vi "MagX Upload File.vi"(2 "Log File":path=path "C:/Data/April_2019/042419/sp0006_042419.tdms", 3 "Lab notebook entry":string, 4 "Append to Wiki":bool, 5 "Add-on storage":T1, 6 "Station":string="Cell_3", 7 "Create Markdown":bool, 8 "error in":errorcluster, 9 "Experiment ID":string, 10 "Log server":string="magx.lanl.gov", 11 "File name":path=path "C:/Data/April_2019/042419/sp0006_042419.tdms") -> (0 "error out":errorcluster)   [LabVIEW 2024]
uses:
  Add-on Storage.ctl
  <vilib>/httpClient/PUTBuffer.vi
  <vilib>/httpClient/PUTFile.vi
  <vilib>/httpClient/LabVIEWHTTPClient.lvlib
panel:
  out "MD response":string
  out "wiki response":string
  out "Time to upload file":dbl format="%#_gs"
  out "File response":string
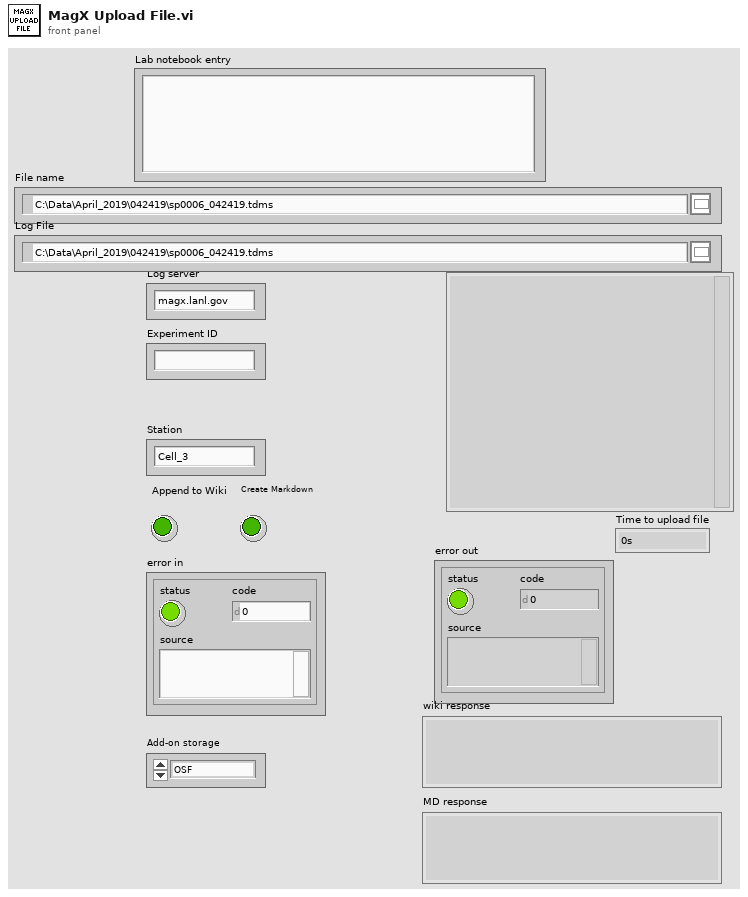
[diagram p1: front panel]
types:
  T1 = typedef "Add-on Storage.ctl" = enum16{"OSF", "OSF - Split", "Google Drive", "Dropbox", "Box"}
  T2 = typedef "LabVIEWHTTPClient.lvlib/ClientHandle.ctl" = refnum<k1>
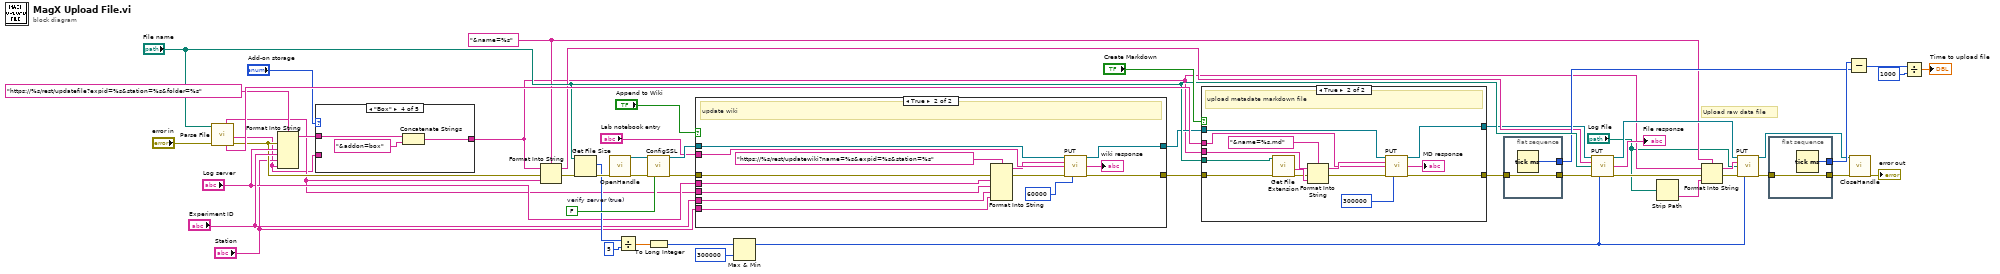
[diagram p0: block diagram]
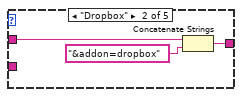
[diagram p3: hidden frame]
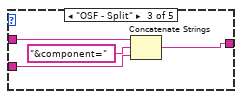
[diagram p4: hidden frame]
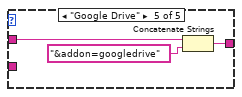
[diagram p5: hidden frame]
diagram:
  w5 = "&name=%s" ("format string")
  w49 = FALSE  # verify server (true)
  # "Upload raw data file"
  n1 = call "Parse File.vi"("error in"="error in", "File name"="File name") -> ("error out"=w27:errorcluster, "Dir 2"=w20:string, "metadata"=w46:string, "File name"=w22:string)  [unwired: 3 in, 3 out]
  n2 = Format Into String(format string="https://%s/rest/updatefile?expid=%s&station=%s&folder=%s", error in=w27, "Log server", "Experiment ID", "Station", w20) -> (resulting string=w25:string)  [unwired: 1 in, 1 out]
  n3 = case shown="\"Box\"" "Add-on storage" {
    tunnel: w25 -> [w53 w56 w60 w63 w66]
    tunnel: [w53 w55 w59 w62 w65] -> w4
    tunnel: w20 -> [_ _ w57 _ _]
    frame "OSF", Default {
    }
    frame "Dropbox" {
      n4 = Concatenate Strings(w56, "&addon=dropbox") -> (w55:string)
    }
    frame "OSF - Split" {
      n5 = Concatenate Strings(w60, "&component=", w57) -> (w59:string)
    }
    frame "Box" {
      n6 = Concatenate Strings(w63, "&addon=box") -> (w62:string)
    }
    frame "Google Drive" {
      n7 = Concatenate Strings(w66, "&addon=googledrive") -> (w65:string)
    }
  }
  n8 = Format Into String(format string=w5, initial string=w4, error in=w27, w22) -> (resulting string=w23:string, error out=w24:errorcluster)
  n9 = Get File Size(file="File name", error in=w24) -> (size (in bytes)=w42:i64, 0:w43:errorcluster)  [unwired: 1 out]
  n10 = call <vilib>:"OpenHandle.vi"("error in (no error)"=w43) -> ("client handle out"=w51:T2, "error out"=w50:errorcluster)  [unwired: 13 in]
  n11 = Divide(x=w42, y=i64 5) -> (x/y=w40:dbl)
  n12 = call <vilib>:"ConfigSSL.vi"("client handle"=w51, "error in (no error)"=w50, "verify server (true)"=w49) -> ("client handle out"=w18:T2, "error out"=w19:errorcluster)  [unwired: 11 in]
  n13 = To Long Integer(number=w40) -> (32bit integer=w39:i32)
  n14 = case shown="True" "Append to Wiki" {
    tunnel: w19 -> [w67 w79]
    tunnel: "Log server" -> [_ w82]
    tunnel: w22 -> [_ w81]
    tunnel: "Experiment ID" -> [_ w80]
    tunnel: w18 -> [w68 w76]
    tunnel: [w68 w75] -> w16
    tunnel: [w67 w74] -> w17
    tunnel: "Lab notebook entry" -> [_ w73]
    tunnel: "Station" -> [_ w69]
    frame False {
    }
    frame True {
      # "update wiki"
      n15 = Format Into String(format string="https://%s/rest/updatewiki?name=%s&expid=%s&station=%s", error in=w79, w82, w81, w80, w69) -> (resulting string=w72:string, error out=w78:errorcluster)  [unwired: 1 in]
      n16 = call-poly <vilib>:"PUT.vi"("client handle"=w76, "url"=w72, "buffer"=w73, "error in (no error)"=w78, "timeout (10000)"=60000) -> ("client handle out"=w75:T2, "body"=→"wiki response":string, "error out"=w74:errorcluster)  [unwired: 7 in, 1 out]
    }
  }
  n17 = Max & Min(x=w39, y=300000) -> (max(x,y)=w1:i32)  [unwired: 1 out]
  n18 = case shown="True" "Create Markdown" {
    tunnel: w16 -> [w84 w98]
    tunnel: "File name" -> [_ w97]
    tunnel: w17 -> [w83 w95]
    tunnel: w46 -> [_ w91]
    tunnel: [w83 w90] -> w15
    tunnel: [w84 w89] -> w14
    tunnel: w4 -> [_ w86]
    frame False {
    }
    frame True {
      # "upload metadate markdown file"
      n19 = call <vilib>:"Get File Extension.vi"("error in (no error)"=w95, "file"=w97) -> ("error out"=w94:errorcluster, "filename without extension"=w96:string)  [unwired: 5 in, 3 out]
      n20 = Format Into String(format string="&name=%s.md", initial string=w86, error in=w94, w96) -> (resulting string=w92:string, error out=w93:errorcluster)
      n21 = call-poly <vilib>:"PUT.vi"("client handle"=w98, "url"=w92, "buffer"=w91, "error in (no error)"=w93, "timeout (10000)"=300000) -> ("client handle out"=w89:T2, "body"=→"MD response":string, "error out"=w90:errorcluster)  [unwired: 7 in, 1 out]
    }
  }
  n22 = flat-sequence {
    tunnel: w15 -> [w100]
    tunnel: [w100] -> w37
    tunnel: [w99] -> w35
    frame #0 {
      n23 = Tick Count (ms)() -> (millisecond timer value=w99:u32)
    }
  }
  n24 = call-poly <vilib>:"PUT.vi"("client handle"=w14, "url"=w23, "file"="File name", "error in (no error)"=w37, "timeout (10000)"=w1) -> ("client handle out"=w10:T2, "body"=→"File response":string, "error out"=w8:errorcluster)  [unwired: 7 in, 1 out]
  n25 = Strip Path(path="Log File") -> (name=w2:string)  [unwired: 1 out]
  n26 = Format Into String(format string=w5, initial string=w4, error in=w8, w2) -> (resulting string=w6:string, error out=w7:errorcluster)
  n27 = call-poly <vilib>:"PUT.vi"("client handle"=w10, "url"=w6, "file"="Log File", "error in (no error)"=w7, "timeout (10000)"=w1) -> ("client handle out"=w9:T2, "error out"=w11:errorcluster)  [unwired: 7 in, 2 out]
  n28 = flat-sequence {
    tunnel: w11 -> [w102]
    tunnel: [w102] -> w13
    tunnel: [w101] -> w36
    frame #0 {
      n29 = Tick Count (ms)() -> (millisecond timer value=w101:u32)
    }
  }
  n30 = Subtract(x=w36, y=w35) -> (x-y=w34:u32)
  n31 = call <vilib>:"CloseHandle.vi"("client handle"=w9, "error in (no error)"=w13) -> ("error out"=→"error out":errorcluster)  [unwired: 13 in]
  n32 = Divide(x=w34, y=u32 1000) -> (x/y=→"Time to upload file":dbl)
